vi "LogFile Part.vi"(8 "as Column":bool, 9 "Länge":i32, 10 "Key":string, 11 "Data":string[][](array[string])) -> (3 "Part Array":string[][](array[string]))   [LabVIEW 2020, in "Linearisierung v2.lvlib" / "SpanEinstellungen.lvlib"]
uses:
  SpanEinstellungen.lvlib
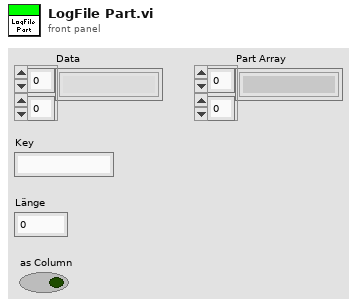
[diagram p1: front panel]
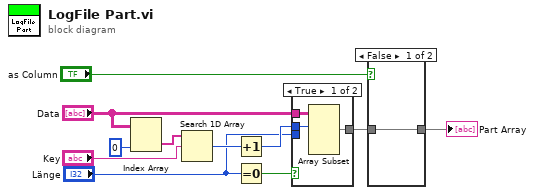
[diagram p0: block diagram]
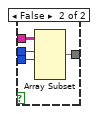
[diagram p2: hidden frame]
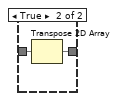
[diagram p3: hidden frame]
diagram:
  n1 = Index Array(array="Data", index (col)=0 ("Deaktivierter Index (Spalte)")) -> (element=w6:string[])  [unwired: 1 in]
  n2 = Search 1D Array(1D array=w6, element="Key") -> (index of element=w9:i32)  [unwired: 1 in]
  n3 = Increment(x=w9) -> (x+1=w10:i32)
  n4 = Equal To 0?(x="Länge") -> (x = 0?=w1:bool)
  n5 = case shown="True" w1 {
    tunnel: w10 -> [w14 w18]
    tunnel: "Data" -> [w13 w17]
    tunnel: "Länge" -> [_ w16]
    tunnel: [w12 w15] -> w5
    frame True {
      n6 = Array Subset(array=w13, index (row)=w14) -> (w12:string[][])  [unwired: 3 in]
    }
    frame False {
      n7 = Array Subset(array=w17, index (row)=w18, length (row)=w16) -> (w15:string[][])  [unwired: 2 in]
    }
  }
  n8 = case shown="False" "as Column" {
    tunnel: w5 -> [w19 w21]
    tunnel: [w19 w20] -> w4
    frame False {
    }
    frame True {
      n9 = Transpose 2D Array(2D array=w21) -> (transposed array=w20:string[][])
    }
  }
  "Part Array" <- w4
